vi "Original Config.vi"(11 "Config File in":refnum<class "Config File.lvclass">) -> (2 "Original Config (as read from the file)":string="{}")   [LabVIEW 2020, in "Config File.lvclass"]
doc: "The original config info as initially read from the config file (as as most recently written by this Config File object)."
uses:
  <vilib>/JDP Science/JSONtext/Config Files/Config File.lvclass
  <vilib>/JDP Science/JSONtext/Config Files/Config File.lvclass/Config File.ctl
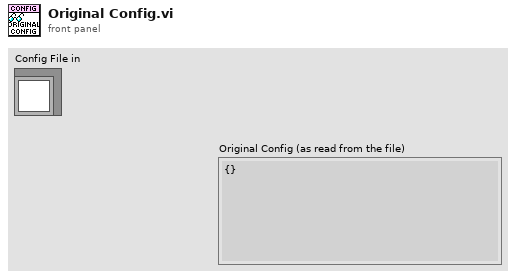
[diagram p1: front panel]
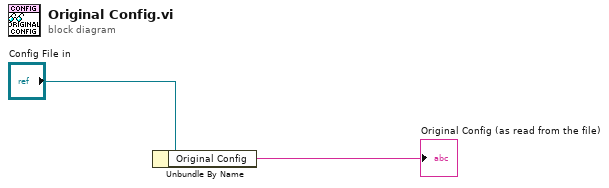
[diagram p0: block diagram]
diagram:
  n1 = Unbundle By Name("Config File in") -> ("Original Config"=→"Original Config (as read from the file)":string)
